vi "Start Request.vi"(10 "error in (no error)":errorcluster, 11 "RequestTraceLog in":refnum<class "RequestTraceLog.lvclass">) -> (2 "error out":errorcluster, 3 "RequestTraceLog out":refnum<class "RequestTraceLog.lvclass">)   [LabVIEW 2020, in "HTTP Server.lvlib" / "RequestTraceLog.lvclass"]
uses:
  RequestTraceLog.lvclass
  RequestTraceLog.lvclass/RequestTraceLog.ctl
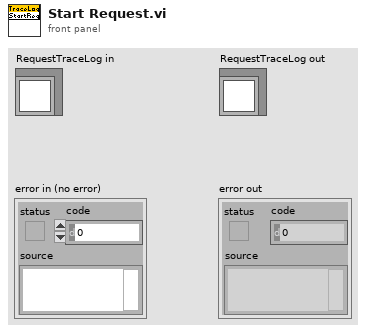
[diagram p1: front panel]
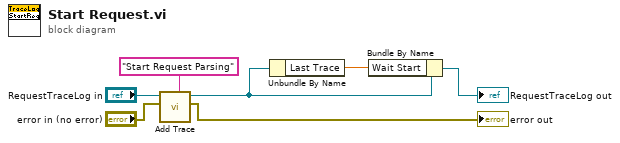
[diagram p0: block diagram]
diagram:
  n1 = call "Add Trace.vi"("Info"="Start Request Parsing", "error in (no error)"="error in (no error)", "RequestTraceLog in"="RequestTraceLog in") -> ("error out"=→"error out":errorcluster, "RequestTraceLog out"=w2:refnum<class "RequestTraceLog.lvclass">)  [unwired: 7 in]
  n2 = Unbundle By Name(w2) -> ("Last Trace"=w1:dbl)
  n3 = Bundle By Name(cluster=w2, "Wait Start"=w1) -> (→"RequestTraceLog out":refnum<class "RequestTraceLog.lvclass">)
